vi "getDataFile.vi"(8 "error in (no error)":errorcluster, 11 "reference in":refnum<class "excelFile.lvclass">) -> (0 "error out":errorcluster, 3 "reference out":refnum<class "excelFile.lvclass">)   [LabVIEW 2015, in "excelFile.lvclass"]
uses:
  excelFile.lvclass
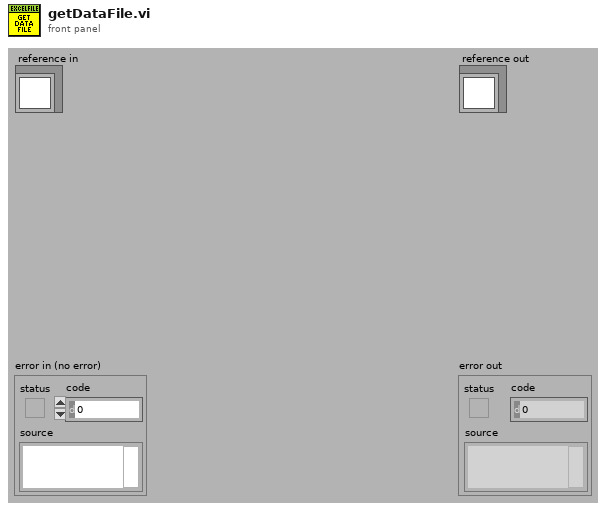
[diagram p1: front panel]
types:
  T1 = typedef "excelFile.lvclass/ObjectAttributesRef.ctl" = refnum<data-value>
  T2 = typedef "excelFile.lvclass/ObjectAttributes.ctl" = cluster{"MyAttribute":dbl, "path":string, "Refnum Excel":cluster{"Excel._Application":refnum<k7>, "Workbooks":refnum<k7>, "Open":refnum<k7>}, "data":string[][][], "fileType":T3, "sheetName":string[]}
  T3 = typedef "excelFile.lvclass/fileType.ctl" = enum16{"database", "CosmedTest PFTSUITE", "CosmedTest OMNIA"}
  T4 = cluster{"Excel._Application":refnum<k7>, "Workbooks":refnum<k7>, "Open":refnum<k7>}
  T5 = cluster{"Excel._Application":refnum<k7>, "Workbooks":refnum<k7>, "Open":refnum<k7>, "Worksheets":refnum<k7>, "Excel._Worksheet":refnum<k7>}
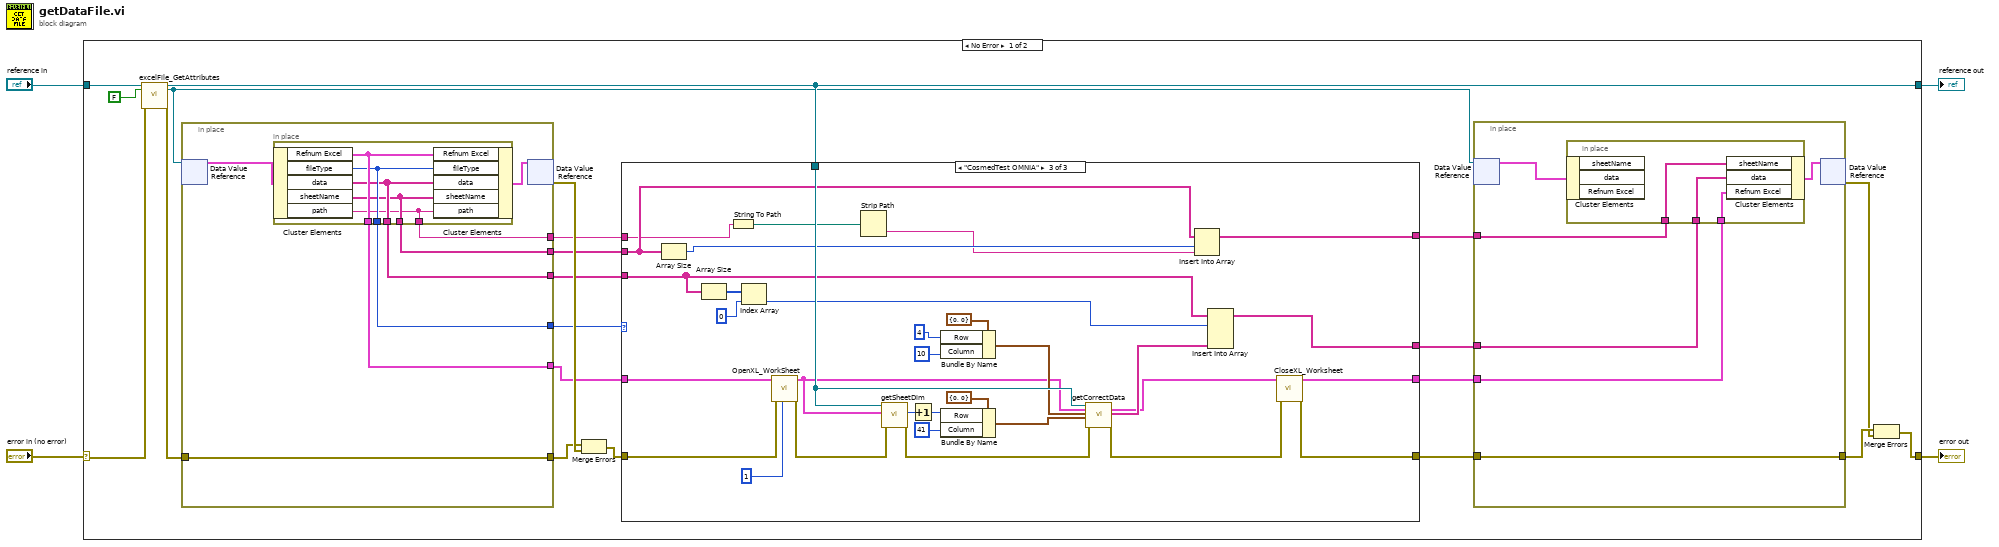
[diagram p0: block diagram]
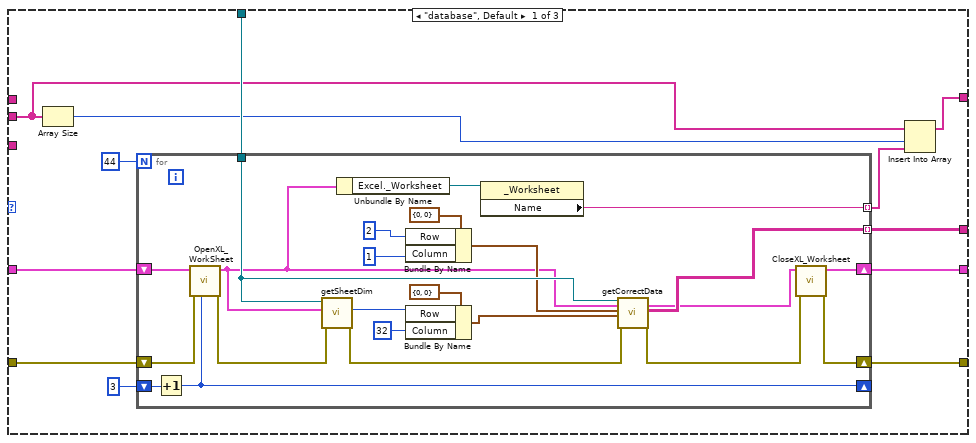
[diagram p2: hidden frame]
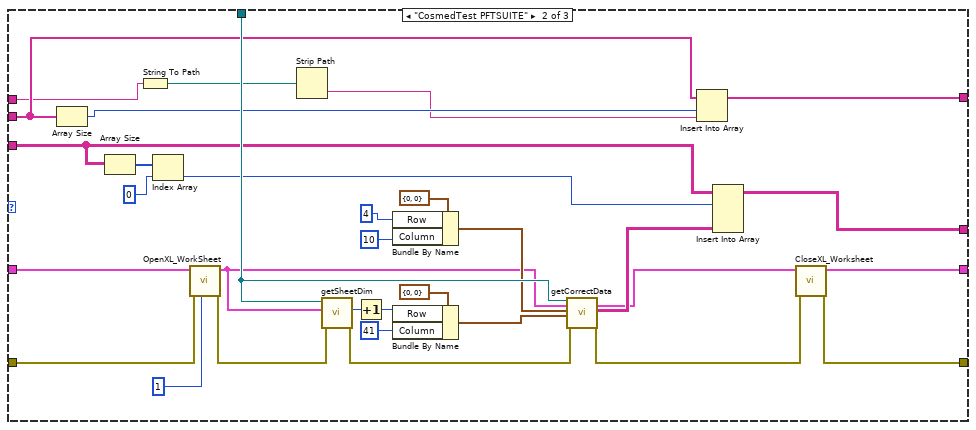
[diagram p3: hidden frame]
diagram:
  n1 = case shown="No Error" "error in (no error)" {
    selector: "error in (no error)" -> [w21 w148]
    tunnel: [w11 w148] -> w3
    tunnel: [w16 w147] -> w1
    tunnel: "reference in" -> [w23 w147]
    frame No Error {
      n2 = call "excelFile_GetAttributes.vi"("reference in"=w23, "return data? (T)"=FALSE, "error in (no error)"=w21) -> ("reference out"=w16:refnum<class "excelFile.lvclass">, "attributes ref"=w14:T1, "error out"=w20:errorcluster)  [unwired: 13 in, 1 out]
      n3 = in-place {
        in-place-border: w20 -> [w139]
        in-place-border: [w139] -> w24
        in-place-border: [w138] -> w17
        in-place-border: [w137] -> w18
        in-place-border: [w136] -> w10
        in-place-border: [w135] -> w9
        in-place-border: [w134] -> w7
        n4 = in-place-dvr #1(w14) -> (w140:T2)  [unwired: 1 out]
        n5 = in-place {
          in-place-border: [w146] -> w138
          in-place-border: [w145] -> w137
          in-place-border: [w144] -> w136
          in-place-border: [w143] -> w135
          in-place-border: [w142] -> w134
          n6 = in-place-cluster #2(w140) -> ("Refnum Excel"=w146:T4, "fileType"=w145:T3, "data"=w144:string[][][], "sheetName"=w143:string[], "path"=w142:string)
          n7 = in-place-cluster #2("Refnum Excel"=w146, "fileType"=w145, "data"=w144, "sheetName"=w143, "path"=w142) -> (w141:T2)
        }
        n8 = in-place-dvr #1(w141) -> (w25:errorcluster)  [unwired: 1 out]
      }
      n9 = Merge Errors(w24, w25) -> (w19:errorcluster)
      n10 = case shown="\"CosmedTest OMNIA\"" w18 {
        tunnel: w19 -> [w46 w101 w133]
        tunnel: [w45 w99 w131] -> w15
        tunnel: w17 -> [w44 w100 w132]
        tunnel: w16 -> [w43 w91 w123]
        tunnel: [w40 w80 w112] -> w6
        tunnel: w10 -> [_ w85 w117]
        tunnel: w9 -> [w37 w78 w110]
        tunnel: [w36 w76 w108] -> w8
        tunnel: w7 -> [_ w75 w107]
        tunnel: [w35 w71 w103] -> w5
        frame "database", Default {
          n11 = Array Size(array=w37) -> (size(s)=w39:i32)
          n12 = for {
            N: 44 -> [_]
            shift-right: [w61] -> w45
            shift-left: w46 -> [w64]
            tunnel: w43 -> [w56]
            tunnel: [w51] -> w40 mode=indexing
            shift-right: [w62] -> w35
            shift-left: w44 -> [w65]
            shift-right: [w57] -> _
            shift-left: 3 -> [w58]
            tunnel: [w48] -> w38 mode=indexing
            n13 = Increment(x=w58) -> (x+1=w57:i32)
            n14 = call <userlib>:"OpenXL_WorkSheet.vi"("Sheet"=w57, "error in (no error)"=w64, "Refnum Cluster In"=w65) -> ("error out"=w63:errorcluster, "Refnum Cluster Out"=w49:T5)  [unwired: 7 in]
            n15 = call "getSheetDim.vi"("error in (no error)"=w63, "Refnum Cluster Out"=w49, "reference in"=w56) -> ("error out"=w53:errorcluster, "rowNumber"=w60:i32)  [unwired: 6 in, 1 out]
            n16 = Unbundle By Name(w49) -> ("Excel._Worksheet"=w50:refnum<k7>)
            n17 = Bundle By Name(cluster=cluster{"Column":i32, "Row":i32} {"Column"=0, "Row"=0} ("Start"), "Row"=2 ("Column"), "Column"=1) -> (w55:cluster{"Column":i32, "Row":i32})
            n18 = Bundle By Name(cluster=cluster{"Column":i32, "Row":i32} {"Column"=0, "Row"=0} ("Start"), "Row"=w60, "Column"=32) -> (w54:cluster{"Column":i32, "Row":i32})
            n19 = property class="_Worksheet"(reference=w50) -> ("Name"=w48:string)  [unwired: 1 in, 2 out]
            n20 = call "getCorrectData.vi"("reference in"=w56, "Refnum Cluster In"=w49, "Start"=w55, "End"=w54, "error in (no error)"=w53) -> ("Refnum Cluster Out"=w47:T5, "data"=w51:string[][], "error out"=w52:errorcluster)  [unwired: 11 in, 1 out]
            n21 = call <userlib>:"CloseXL_Worksheet.vi"("error in (no error)"=w52, "Refnum Cluster In"=w47) -> ("error out"=w61:errorcluster, "Refnum Cluster Out"=w62:T4)  [unwired: 8 in]
          }
          n22 = Insert Into Array(array=w37, index=w39, new element=w38) -> (w36:string[])
        }
        frame "CosmedTest PFTSUITE" {
          n23 = Array Size(array=w78) -> (size(s)=w77:i32)
          n24 = Array Size(array=w85) -> (size(s)=w84:i32[])
          n25 = String To Path(string=w75) -> (path=w74:path)
          n26 = Index Array(array=w84, index=0) -> (element=w82:i32)
          n27 = call <userlib>:"OpenXL_WorkSheet.vi"("Sheet"=1, "error in (no error)"=w101, "Refnum Cluster In"=w100) -> ("error out"=w94:errorcluster, "Refnum Cluster Out"=w79:T5)  [unwired: 7 in]
          n28 = Strip Path(path=w74) -> (name=w73:string)  [unwired: 1 out]
          n29 = call "getSheetDim.vi"("error in (no error)"=w94, "Refnum Cluster Out"=w79, "reference in"=w91) -> ("error out"=w87:errorcluster, "rowNumber"=w93:i32)  [unwired: 6 in, 1 out]
          n30 = Increment(x=w93) -> (x+1=w72:i32)
          n31 = Bundle By Name(cluster=cluster{"Column":i32, "Row":i32} {"Column"=0, "Row"=0} ("Start"), "Row"=4 ("Column"), "Column"=10) -> (w89:cluster{"Column":i32, "Row":i32})
          n32 = Bundle By Name(cluster=cluster{"Column":i32, "Row":i32} {"Column"=0, "Row"=0} ("Start"), "Row"=w72, "Column"=41) -> (w88:cluster{"Column":i32, "Row":i32})
          n33 = call "getCorrectData.vi"("reference in"=w91, "Refnum Cluster In"=w79, "Start"=w89, "End"=w88, "error in (no error)"=w87) -> ("Refnum Cluster Out"=w70:T5, "data"=w81:string[][], "error out"=w86:errorcluster)  [unwired: 11 in, 1 out]
          n34 = Insert Into Array(array=w78, index=w77, new element=w73) -> (w76:string[])
          n35 = Insert Into Array(array=w85, index (dim 0)=w82, new element=w81) -> (w80:string[][][])  [unwired: 2 in]
          n36 = call <userlib>:"CloseXL_Worksheet.vi"("error in (no error)"=w86, "Refnum Cluster In"=w70) -> ("error out"=w99:errorcluster, "Refnum Cluster Out"=w71:T4)  [unwired: 8 in]
        }
        frame "CosmedTest OMNIA" {
          n37 = Array Size(array=w110) -> (size(s)=w109:i32)
          n38 = Array Size(array=w117) -> (size(s)=w116:i32[])
          n39 = String To Path(string=w107) -> (path=w106:path)
          n40 = Index Array(array=w116, index=0) -> (element=w114:i32)
          n41 = call <userlib>:"OpenXL_WorkSheet.vi"("Sheet"=1, "error in (no error)"=w133, "Refnum Cluster In"=w132) -> ("error out"=w126:errorcluster, "Refnum Cluster Out"=w111:T5)  [unwired: 7 in]
          n42 = Strip Path(path=w106) -> (name=w105:string)  [unwired: 1 out]
          n43 = call "getSheetDim.vi"("error in (no error)"=w126, "Refnum Cluster Out"=w111, "reference in"=w123) -> ("error out"=w119:errorcluster, "rowNumber"=w125:i32)  [unwired: 6 in, 1 out]
          n44 = Increment(x=w125) -> (x+1=w104:i32)
          n45 = Bundle By Name(cluster=cluster{"Column":i32, "Row":i32} {"Column"=0, "Row"=0} ("Start"), "Row"=4 ("Column"), "Column"=10) -> (w121:cluster{"Column":i32, "Row":i32})
          n46 = Bundle By Name(cluster=cluster{"Column":i32, "Row":i32} {"Column"=0, "Row"=0} ("Start"), "Row"=w104, "Column"=41) -> (w120:cluster{"Column":i32, "Row":i32})
          n47 = call "getCorrectData.vi"("reference in"=w123, "Refnum Cluster In"=w111, "Start"=w121, "End"=w120, "error in (no error)"=w119) -> ("Refnum Cluster Out"=w102:T5, "data"=w113:string[][], "error out"=w118:errorcluster)  [unwired: 11 in, 1 out]
          n48 = Insert Into Array(array=w110, index=w109, new element=w105) -> (w108:string[])
          n49 = Insert Into Array(array=w117, index (dim 0)=w114, new element=w113) -> (w112:string[][][])  [unwired: 2 in]
          n50 = call <userlib>:"CloseXL_Worksheet.vi"("error in (no error)"=w118, "Refnum Cluster In"=w102) -> ("error out"=w131:errorcluster, "Refnum Cluster Out"=w103:T4)  [unwired: 8 in]
        }
      }
      n51 = in-place {
        in-place-border: w15 -> [w29]
        in-place-border: [w29] -> w13
        in-place-border: w6 -> [w28]
        in-place-border: w8 -> [w27]
        in-place-border: w5 -> [w26]
        n52 = in-place-dvr #3(w14) -> (w30:T2)  [unwired: 1 out]
        n53 = in-place {
          in-place-border: w28 -> [w34]
          in-place-border: w27 -> [w33]
          in-place-border: w26 -> [w32]
          n54 = in-place-cluster #4(w30) -> ()  [unwired: 3 out]
          n55 = in-place-cluster #4("sheetName"=w33, "data"=w34, "Refnum Excel"=w32) -> (w31:T2)
        }
        n56 = in-place-dvr #3(w31) -> (w12:errorcluster)  [unwired: 1 out]
      }
      n57 = Merge Errors(w13, w12) -> (w11:errorcluster)
    }
    frame Error {
    }
  }
  "error out" <- w3
  "reference out" <- w1
